vi "Indicator Type.vi"(11 "Indicator in":refnum<class "Indicator.lvclass">) -> (2 "Indicator Type":string)   [LabVIEW 2020, in "VolatusGUI.lvlib" / "Indicator.lvclass"]
uses:
  Indicator.lvclass
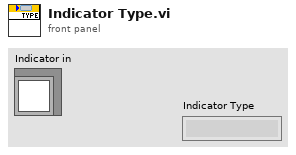
[diagram p1: front panel]
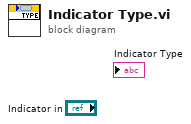
[diagram p0: block diagram]
diagram:
